vi "executeKeeperPlay.vi"(8 "error in (no error)":errorcluster, 11 "Game in":refnum<class "Game.lvclass">) -> (0 "error out":errorcluster, 3 "Game out":refnum<class "Game.lvclass">)   [LabVIEW 2023, in "Game.lvclass"]
uses:
  Game.lvclass
  Game.lvclass/Game.ctl
  Team_class/Team.lvclass/Team.ctl
  Playbook_class/Playbook.lvclass/Playbook.ctl
  TestPlay_class/TestPlay.lvclass/TestPlay.ctl
  TimeoutPlay_class/TimeoutPlay.lvclass/TimeoutPlay.ctl
  ZigZagPlay_class/ZigZagPlay.lvclass/ZigZagPlay.ctl
  HaltPlay_class/HaltPlay.lvclass/HaltPlay.ctl
  Playbook_class/Read keeper_plays.vi
  TestPlay_class/Read Roles.vi
  TimeoutPlay_class/Read Roles.vi
  ZigZagPlay_class/Read Roles.vi
  HaltPlay_class/Read Roles.vi
  Read KeeperTeam.vi
  Team_class/Read RobotRef.vi
  Team_class/Read KeeperPlay.vi
  Team_class/Write RobotRef.vi
  Write KeeperTeam.vi
  Ally_class/Ally.lvclass
  Playbook_class/Playbook.lvclass
  Robot_class/Robot.lvclass
  Play_class/Play.lvclass
  TestPlay_class/TestPlay.lvclass
  HaltPlay_class/HaltPlay.lvclass
  KeeperPlay_class/KeeperPlay.lvclass
  TimeoutPlay_class/TimeoutPlay.lvclass
  ZigZagPlay_class/ZigZagPlay.lvclass
  GoToPlay_class/GoToPlay.lvclass
  TestRole_class/TestRole.lvclass
  Role_class/Role.lvclass
  KeeperRole_class/KeeperRole.lvclass
  TimeoutRole_class/TimeoutRole.lvclass
  ZigZagRole_class/ZigZagRole.lvclass
  HaltRole_class/HaltRole.lvclass
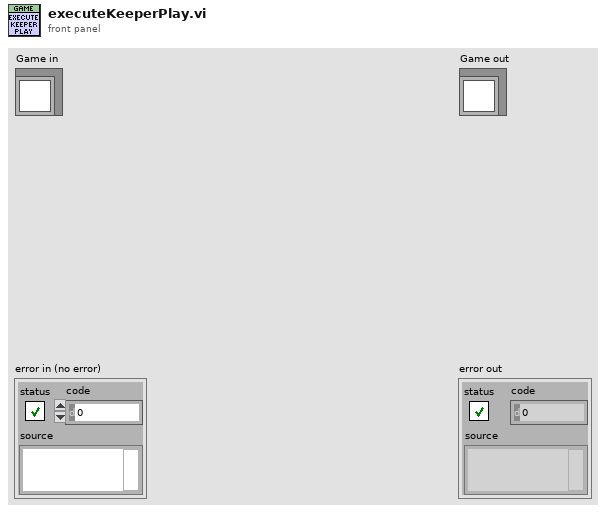
[diagram p1: front panel]
types:
  T1 = typedef "KeeperPlay.ctl" = enum16{"ZigZag", "Goto", "NormalGame", "KeeperPlay", "Halt", "Timeout", "PenaltyEnemy", "TestPlay"}
  T2 = typedef "keeper_plays.ctl" = cluster{"Play":refnum<class "Play.lvclass">, "TestPlay":refnum<class "TestPlay.lvclass">, "HaltPlay":refnum<class "HaltPlay.lvclass">, "KeeperPlay":refnum<class "KeeperPlay.lvclass">, "TimeoutPlay":refnum<class "TimeoutPlay.lvclass">, "ZigZagPlay":refnum<class "ZigZagPlay.lvclass">, "GoToPlay":refnum<class "GoToPlay.lvclass">}
  T3 = cluster{"TestRole 1":refnum<class "TestRole.lvclass">, "Role":refnum<class "Role.lvclass">, "TestRole 2":refnum<class "TestRole.lvclass">, "TestRole 3":refnum<class "TestRole.lvclass">}
  T4 = cluster{"KeeperRole":refnum<class "KeeperRole.lvclass">}
  T5 = cluster{"TimeoutRole 1":refnum<class "TimeoutRole.lvclass">, "TimeoutRole 2":refnum<class "TimeoutRole.lvclass">, "TimeoutRole 3":refnum<class "TimeoutRole.lvclass">, "TimeoutRole 4":refnum<class "TimeoutRole.lvclass">, "TimeoutRole 5":refnum<class "TimeoutRole.lvclass">, "TimeoutRole 6":refnum<class "TimeoutRole.lvclass">}
  T6 = cluster{"ZigZagRole":refnum<class "ZigZagRole.lvclass">}
  T7 = cluster{"HaltRole 1":refnum<class "HaltRole.lvclass">, "HaltRole 2":refnum<class "HaltRole.lvclass">, "HaltRole 3":refnum<class "HaltRole.lvclass">, "HaltRole 4":refnum<class "HaltRole.lvclass">, "HaltRole 5":refnum<class "HaltRole.lvclass">, "HaltRole 6":refnum<class "HaltRole.lvclass">}
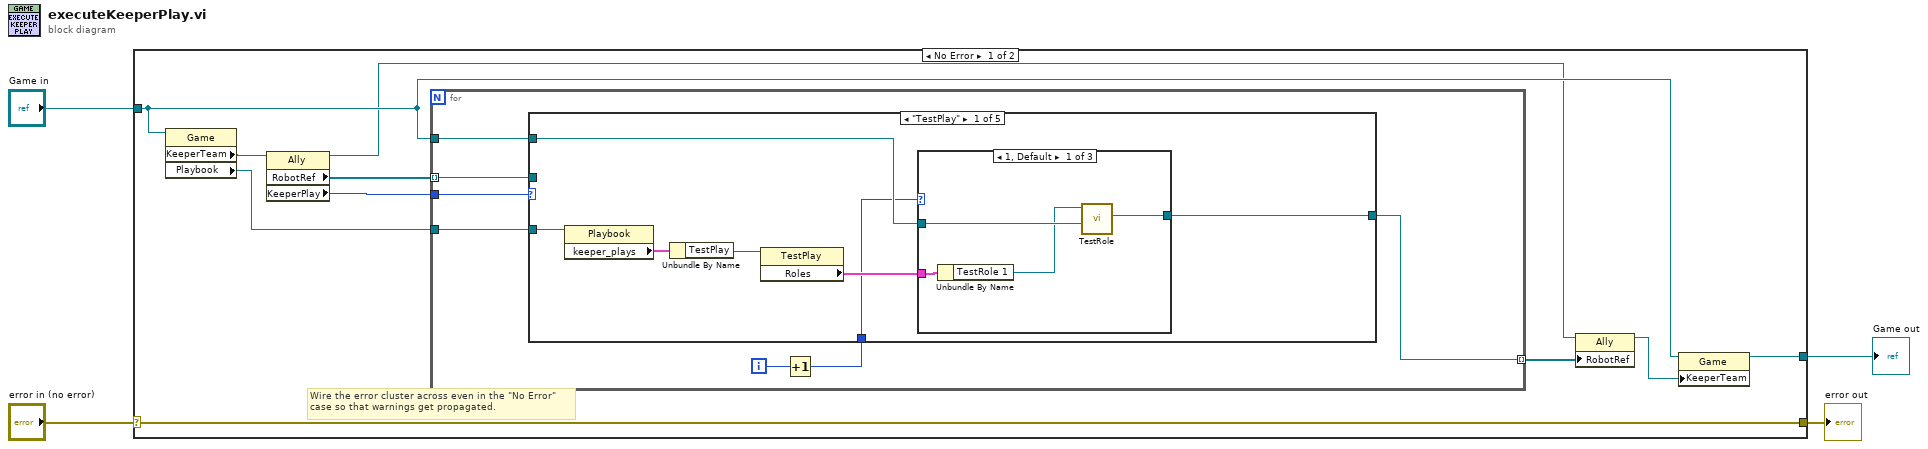
[diagram p0: block diagram]
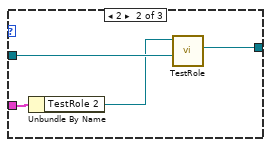
[diagram p2: hidden frame]
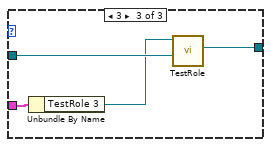
[diagram p3: hidden frame]
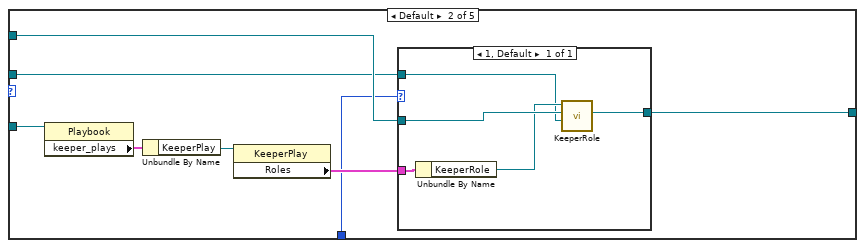
[diagram p4: hidden frame]
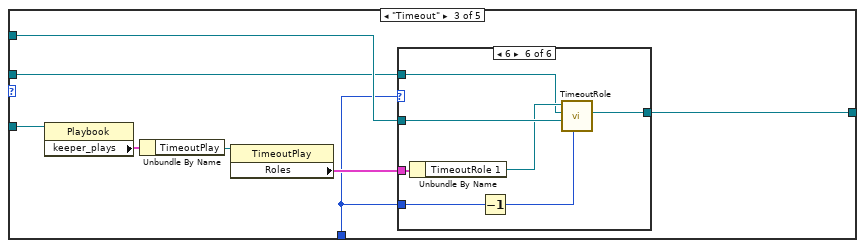
[diagram p5: hidden frame]
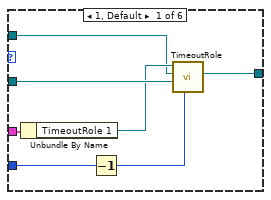
[diagram p6: hidden frame]
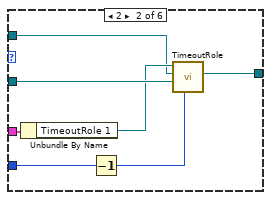
[diagram p7: hidden frame]
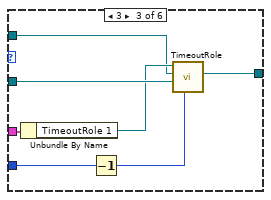
[diagram p8: hidden frame]
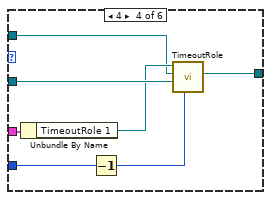
[diagram p9: hidden frame]
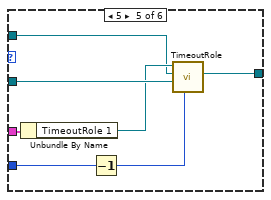
[diagram p10: hidden frame]
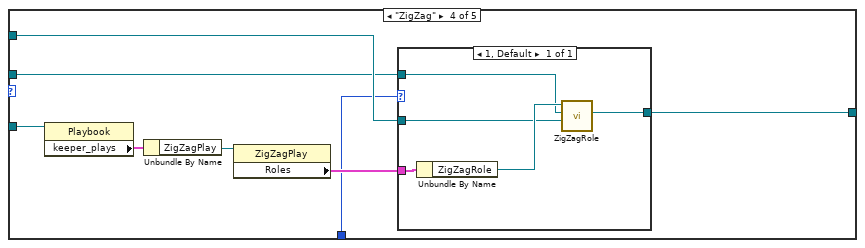
[diagram p11: hidden frame]
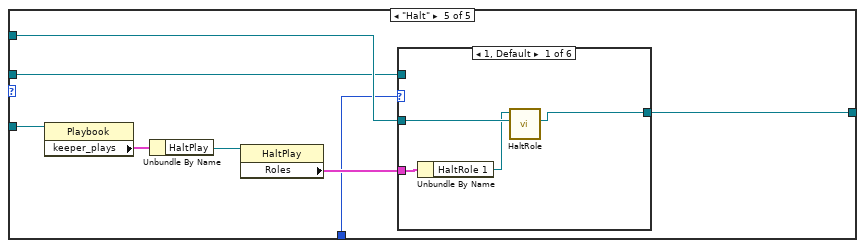
[diagram p12: hidden frame]
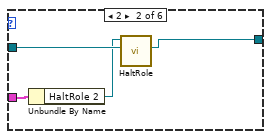
[diagram p13: hidden frame]
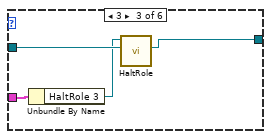
[diagram p14: hidden frame]
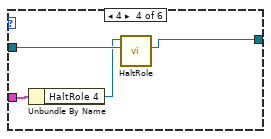
[diagram p15: hidden frame]
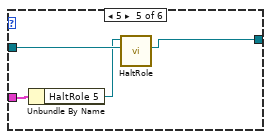
[diagram p16: hidden frame]
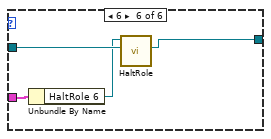
[diagram p17: hidden frame]
diagram:
  n1 = case shown="No Error" "error in (no error)" {
    selector: "error in (no error)" -> [w14 w150]
    tunnel: [w14 w150] -> w3
    tunnel: [w7 w149] -> w1
    tunnel: "Game in" -> [w9 w149]
    frame No Error {
      # "Wire the error cluster across even in the \"No Error\"\ncase so that warnings get propagated."
      n2 = property class="Game"(reference=w9) -> ("KeeperTeam"=w13:refnum<class "Ally.lvclass">, "Playbook"=w10:refnum<class "Playbook.lvclass">)  [unwired: 1 in, 2 out]
      n3 = property class="Ally"(reference=w13) -> (reference out=w8:refnum<class "Ally.lvclass">, "RobotRef"=w12:refnum<class "Robot.lvclass">[], "KeeperPlay"=w11:T1)  [unwired: 1 in, 1 out]
      n4 = for {
        tunnel: w12 -> [w15] mode=indexing
        tunnel: w11 -> [w21]
        tunnel: w10 -> [w20]
        tunnel: w9 -> [w19]
        tunnel: [w18] -> w5 mode=indexing
        i -> [w17]
        n5 = Increment(x=w17) -> (x+1=w16:i32)
        n6 = case shown="\"TestPlay\"" w21 {
          tunnel: w20 -> [w28 w48 w61 w111 w124]
          tunnel: w19 -> [w24 w44 w57 w107 w120]
          tunnel: [w23 w43 w56 w106 w119] -> w18
          tunnel: w16 -> [w22 w42 w54 w105 w118]
          tunnel: w15 -> [_ w41 w55 w104 w117]
          frame "TestPlay" {
            n7 = property class="Playbook"(reference=w28) -> ("keeper_plays"=w27:T2)  [unwired: 1 in, 2 out]
            n8 = Unbundle By Name(w27) -> ("TestPlay"=w26:refnum<class "TestPlay.lvclass">)
            n9 = property class="TestPlay"(reference=w26) -> ("Roles"=w25:T3)  [unwired: 1 in, 2 out]
            n10 = case shown="1, Default" w22 {
              tunnel: w25 -> [w32 w36 w40]
              tunnel: w24 -> [w31 w35 w39]
              tunnel: [w30 w34 w38] -> w23
              frame 1, Default {
                n11 = Unbundle By Name(w32) -> ("TestRole 1"=w29:refnum<class "TestRole.lvclass">)
                n12 = call-dynamic "TestRole.vi"("Game in"=w31, "TestRole in"=w29) -> ("Robot out"=w30:refnum<class "Robot.lvclass">)  [unwired: 6 in, 3 out]
              }
              frame 2 {
                n13 = Unbundle By Name(w36) -> ("TestRole 2"=w33:refnum<class "TestRole.lvclass">)
                n14 = call-dynamic "TestRole.vi"("Game in"=w35, "TestRole in"=w33) -> ("Robot out"=w34:refnum<class "Robot.lvclass">)  [unwired: 6 in, 3 out]
              }
              frame 3 {
                n15 = Unbundle By Name(w40) -> ("TestRole 3"=w37:refnum<class "TestRole.lvclass">)
                n16 = call-dynamic "TestRole.vi"("Game in"=w39, "TestRole in"=w37) -> ("Robot out"=w38:refnum<class "Robot.lvclass">)  [unwired: 6 in, 3 out]
              }
            }
          }
          frame Default {
            n17 = property class="Playbook"(reference=w48) -> ("keeper_plays"=w47:T2)  [unwired: 1 in, 2 out]
            n18 = Unbundle By Name(w47) -> ("KeeperPlay"=w46:refnum<class "KeeperPlay.lvclass">)
            n19 = property class="KeeperPlay"(reference=w46) -> ("Roles"=w45:T4)  [unwired: 1 in, 2 out]
            n20 = case shown="1, Default" w42 {
              tunnel: w45 -> [w53]
              tunnel: w44 -> [w52]
              tunnel: [w51] -> w43
              tunnel: w41 -> [w49]
              frame 1, Default {
                n21 = Unbundle By Name(w53) -> ("KeeperRole"=w50:refnum<class "KeeperRole.lvclass">)
                n22 = call "KeeperRole.vi"("Robot in"=w49, "Game in"=w52, "KeeperRole in"=w50) -> ("Robot out"=w51:refnum<class "Robot.lvclass">)  [unwired: 6 in, 2 out]
              }
            }
          }
          frame "Timeout" {
            n23 = property class="Playbook"(reference=w61) -> ("keeper_plays"=w60:T2)  [unwired: 1 in, 2 out]
            n24 = Unbundle By Name(w60) -> ("TimeoutPlay"=w59:refnum<class "TimeoutPlay.lvclass">)
            n25 = property class="TimeoutPlay"(reference=w59) -> ("Roles"=w58:T5)  [unwired: 1 in, 2 out]
            n26 = case shown="6" w54 {
              tunnel: w58 -> [w68 w75 w82 w89 w96 w103]
              tunnel: w57 -> [w67 w74 w81 w88 w95 w102]
              tunnel: [w66 w73 w80 w87 w94 w101] -> w56
              tunnel: w55 -> [w64 w71 w78 w85 w92 w99]
              tunnel: w54 -> [w62 w69 w76 w83 w90 w97]
              frame 1, Default {
                n27 = Unbundle By Name(w68) -> ("TimeoutRole 1"=w65:refnum<class "TimeoutRole.lvclass">)
                n28 = Decrement(x=w62) -> (x-1=w63:i32)
                n29 = call-dynamic "TimeoutRole.vi"("robot index in array"=w63, "Game in"=w67, "Robot in"=w64, "TimeoutRole in"=w65) -> ("Robot out"=w66:refnum<class "Robot.lvclass">)  [unwired: 4 in, 3 out]
              }
              frame 2 {
                n30 = Unbundle By Name(w75) -> ("TimeoutRole 1"=w72:refnum<class "TimeoutRole.lvclass">)
                n31 = Decrement(x=w69) -> (x-1=w70:i32)
                n32 = call-dynamic "TimeoutRole.vi"("robot index in array"=w70, "Game in"=w74, "Robot in"=w71, "TimeoutRole in"=w72) -> ("Robot out"=w73:refnum<class "Robot.lvclass">)  [unwired: 4 in, 3 out]
              }
              frame 3 {
                n33 = Unbundle By Name(w82) -> ("TimeoutRole 1"=w79:refnum<class "TimeoutRole.lvclass">)
                n34 = Decrement(x=w76) -> (x-1=w77:i32)
                n35 = call-dynamic "TimeoutRole.vi"("robot index in array"=w77, "Game in"=w81, "Robot in"=w78, "TimeoutRole in"=w79) -> ("Robot out"=w80:refnum<class "Robot.lvclass">)  [unwired: 4 in, 3 out]
              }
              frame 4 {
                n36 = Unbundle By Name(w89) -> ("TimeoutRole 1"=w86:refnum<class "TimeoutRole.lvclass">)
                n37 = Decrement(x=w83) -> (x-1=w84:i32)
                n38 = call-dynamic "TimeoutRole.vi"("robot index in array"=w84, "Game in"=w88, "Robot in"=w85, "TimeoutRole in"=w86) -> ("Robot out"=w87:refnum<class "Robot.lvclass">)  [unwired: 4 in, 3 out]
              }
              frame 5 {
                n39 = Unbundle By Name(w96) -> ("TimeoutRole 1"=w93:refnum<class "TimeoutRole.lvclass">)
                n40 = Decrement(x=w90) -> (x-1=w91:i32)
                n41 = call-dynamic "TimeoutRole.vi"("robot index in array"=w91, "Game in"=w95, "Robot in"=w92, "TimeoutRole in"=w93) -> ("Robot out"=w94:refnum<class "Robot.lvclass">)  [unwired: 4 in, 3 out]
              }
              frame 6 {
                n42 = Unbundle By Name(w103) -> ("TimeoutRole 1"=w100:refnum<class "TimeoutRole.lvclass">)
                n43 = Decrement(x=w97) -> (x-1=w98:i32)
                n44 = call-dynamic "TimeoutRole.vi"("robot index in array"=w98, "Game in"=w102, "Robot in"=w99, "TimeoutRole in"=w100) -> ("Robot out"=w101:refnum<class "Robot.lvclass">)  [unwired: 4 in, 3 out]
              }
            }
          }
          frame "ZigZag" {
            n45 = property class="Playbook"(reference=w111) -> ("keeper_plays"=w110:T2)  [unwired: 1 in, 2 out]
            n46 = Unbundle By Name(w110) -> ("ZigZagPlay"=w109:refnum<class "ZigZagPlay.lvclass">)
            n47 = property class="ZigZagPlay"(reference=w109) -> ("Roles"=w108:T6)  [unwired: 1 in, 2 out]
            n48 = case shown="1, Default" w105 {
              tunnel: w108 -> [w116]
              tunnel: w107 -> [w113]
              tunnel: [w112] -> w106
              tunnel: w104 -> [w114]
              frame 1, Default {
                n49 = Unbundle By Name(w116) -> ("ZigZagRole"=w115:refnum<class "ZigZagRole.lvclass">)
                n50 = call-dynamic "ZigZagRole.vi"("Game in"=w113, "Robot in"=w114, "ZigZagRole in"=w115) -> ("Robot out"=w112:refnum<class "Robot.lvclass">)  [unwired: 5 in, 3 out]
              }
            }
          }
          frame "Halt" {
            n51 = property class="Playbook"(reference=w124) -> ("keeper_plays"=w123:T2)  [unwired: 1 in, 2 out]
            n52 = Unbundle By Name(w123) -> ("HaltPlay"=w122:refnum<class "HaltPlay.lvclass">)
            n53 = property class="HaltPlay"(reference=w122) -> ("Roles"=w121:T7)  [unwired: 1 in, 2 out]
            n54 = case shown="1, Default" w118 {
              tunnel: w121 -> [w128 w132 w136 w140 w144 w148]
              tunnel: w120 -> [w127 w131 w135 w139 w143 w147]
              tunnel: [w125 w129 w133 w137 w141 w145] -> w119
              tunnel: w117 -> [_ _ _ _ _ _]
              frame 1, Default {
                n55 = Unbundle By Name(w128) -> ("HaltRole 1"=w126:refnum<class "HaltRole.lvclass">)
                n56 = call "HaltRole.vi"("Game in"=w127, "HaltRole in"=w126) -> ("Robot out"=w125:refnum<class "Robot.lvclass">)  [unwired: 6 in, 3 out]
              }
              frame 2 {
                n57 = Unbundle By Name(w132) -> ("HaltRole 2"=w130:refnum<class "HaltRole.lvclass">)
                n58 = call "HaltRole.vi"("Game in"=w131, "HaltRole in"=w130) -> ("Robot out"=w129:refnum<class "Robot.lvclass">)  [unwired: 6 in, 3 out]
              }
              frame 3 {
                n59 = Unbundle By Name(w136) -> ("HaltRole 3"=w134:refnum<class "HaltRole.lvclass">)
                n60 = call "HaltRole.vi"("Game in"=w135, "HaltRole in"=w134) -> ("Robot out"=w133:refnum<class "Robot.lvclass">)  [unwired: 6 in, 3 out]
              }
              frame 4 {
                n61 = Unbundle By Name(w140) -> ("HaltRole 4"=w138:refnum<class "HaltRole.lvclass">)
                n62 = call "HaltRole.vi"("Game in"=w139, "HaltRole in"=w138) -> ("Robot out"=w137:refnum<class "Robot.lvclass">)  [unwired: 6 in, 3 out]
              }
              frame 5 {
                n63 = Unbundle By Name(w144) -> ("HaltRole 5"=w142:refnum<class "HaltRole.lvclass">)
                n64 = call "HaltRole.vi"("Game in"=w143, "HaltRole in"=w142) -> ("Robot out"=w141:refnum<class "Robot.lvclass">)  [unwired: 6 in, 3 out]
              }
              frame 6 {
                n65 = Unbundle By Name(w148) -> ("HaltRole 6"=w146:refnum<class "HaltRole.lvclass">)
                n66 = call "HaltRole.vi"("Game in"=w147, "HaltRole in"=w146) -> ("Robot out"=w145:refnum<class "Robot.lvclass">)  [unwired: 6 in, 3 out]
              }
            }
          }
        }
      }
      n67 = property class="Ally"(reference=w8, "RobotRef"=w5) -> (reference out=w6:refnum<class "Ally.lvclass">)  [unwired: 1 in, 1 out]
      n68 = property class="Game"(reference=w9, "KeeperTeam"=w6) -> (reference out=w7:refnum<class "Game.lvclass">)  [unwired: 1 in, 1 out]
    }
    frame Error {
    }
  }
  "error out" <- w3
  "Game out" <- w1
